vi "Create LogRecord.vi"(8 "error in":errorcluster, 9 "Error to Log":errorcluster, 10 "Message":string, 11 "Level":T1) -> (0 "error out":errorcluster, 3 "LogRecord out":refnum<class "LogRecord.lvclass">)   [LabVIEW 2020, in "hse-logger.lvlib" / "LogRecord.lvclass"]
doc: "Creates and initilizes a new LogRecord object.\n\n____\nHAMPEL SOFTWARE ENGINEERING v2.0.6 (2021-04-15 11:38)"
uses:
  LogRecord.lvclass
  LogLevel.ctl
  hse-logger.lvlib
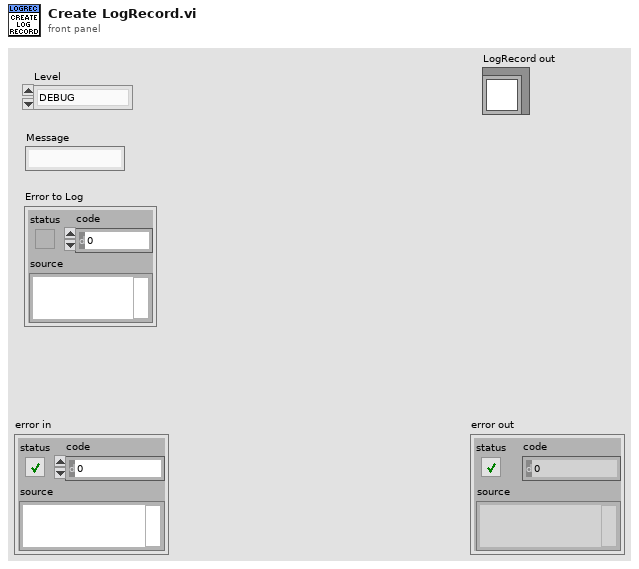
[diagram p1: front panel]
types:
  T1 = typedef "hse-logger.lvlib/LogLevel.ctl" = enum16{"DEBUG", "INFO", "WARNING", "ERROR", "CRITICAL"}
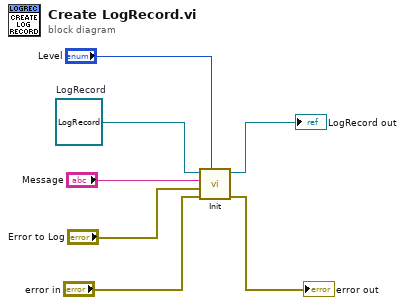
[diagram p0: block diagram]
diagram:
  w2 = refnum<class "LogRecord.lvclass"> refnum  # LogRecord
  n1 = call-dynamic "Init.vi"("Level"="Level", "error in"="error in", "Error to Log"="Error to Log", "Message"="Message", "LogRecord in"=w2) -> ("error out"=→"error out":errorcluster, "LogRecord out"=→"LogRecord out":refnum<class "LogRecord.lvclass">)  [unwired: 5 in]
